vi "Get E2E node ref from UID.vi"(8 "error in (no error)":errorcluster, 11 "UID":string) -> (0 "error out":errorcluster, 3 "E2E editor node ref":refnum<data-value>)   [LabVIEW 2015, in "E2E Tag Exchange editor node.lvclass"]
uses:
  E2E Tag Exchange editor node.lvclass
  Node LUT/Command.ctl
  Node LUT/Node LUT.lvlib
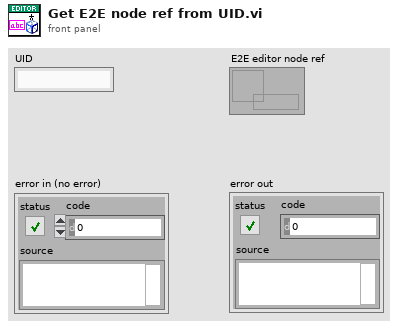
[diagram p1: front panel]
types:
  T1 = typedef "Node LUT.lvlib/Command.ctl" = enum16{"Initialize", "Add Node", "Remove Node", "Node Ref from UID", "List Nodes"}
  T2 = typedef "NISE_CEF_Node.lvclass/NodeRef.ctl" = refnum<data-value>
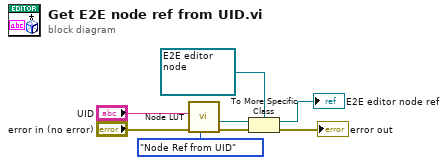
[diagram p0: block diagram]
diagram:
  n1 = call "Node LUT.vi"("Command"=Command."Node Ref from UID", "error in"="error in (no error)", "UID"="UID") -> ("error out"=w6:errorcluster, "node ref"=w3:T2)  [unwired: 5 in, 2 out]
  n2 = To More Specific Class(target class=refnum<data-value> refnum, reference=w3, error in=w6) -> (specific class reference=→"E2E editor node ref":refnum<data-value>, error out=→"error out":errorcluster)
